vi "Create Data Folder.vi"(8 "error in (no error)":errorcluster) -> (0 "error out":errorcluster, 3 "Data path":path)   [LabVIEW 2018]
doc: "Base folder for all xml settings"
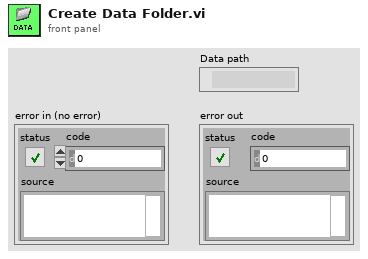
[diagram p1: front panel]
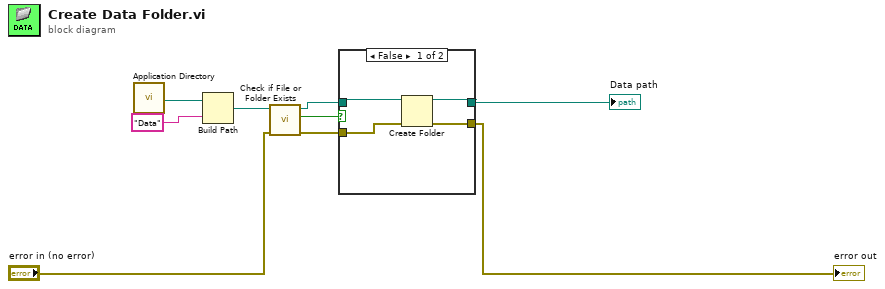
[diagram p0: block diagram]
diagram:
  n1 = call <vilib>:"Application Directory.vi"() -> ("Application Directory"=w1:path)
  n2 = Build Path(base path=w1, name or relative path="Data") -> (appended path=w3:path)
  n3 = call <vilib>:"Check if File or Folder Exists.vi"("error in (no error)"="error in (no error)", "path"=w3) -> ("error out"=w6:errorcluster, "file or folder exists?"=w4:bool, "dup path"=w5:path)  [unwired: 7 in]
  n4 = case shown="False" w4 {
    tunnel: w5 -> [w13 w15]
    tunnel: w6 -> [w12 w14]
    tunnel: [w11 w15] -> w9
    tunnel: [w10 w14] -> w8
    frame False {
      n5 = Create Folder(path (use dialog)=w13, error in=w12) -> (created path=w11:path, error out=w10:errorcluster)  [unwired: 1 in, 1 out]
    }
    frame True {
    }
  }
  "Data path" <- w9
  "error out" <- w8
